vi "pp3_log_sessionParameters.vi"(10 "queue in":refnum<queue>) -> (2 "queue out":refnum<queue>)   [LabVIEW 2013]
uses:
  CTL_pp3c_SessionParam.ctl
panel:
  in  "Session parameters":T1={"Log File Directory Root"=path "E:/Data/SPP.Coulb1", "Subject Name"="SPP074", "Tone repeat (ms)"=0, "Habit tr0 (s)"=180, "ITI min\n(s)"=6, "ITI max\n(s)"=16, "Stay \n(s)"=3, "Run"=TRUE, "Jump time\n(s)"=4, "Start trial"=0, "Log File Directory"=path "E:/Data/SPP.Coulb1/SPP074/161224/161555", "Shock \ndur (s)"=6, "Pre click \n(V)"=0.1, "Click\ndel (s)"=1.0, "Reward CR"=FALSE} {"Click\ndel (s)" min=0.0 step=1.0; "Pre click \n(V)" min=0.0 max=1.0 step=1.0; "Shock \ndur (s)" min=0 step=1; "Stay \n(s)" min=0 step=1; "Start trial" step=1; "Jump time\n(s)" min=0 step=1; "Tone repeat (ms)" min=0 max=1000 step=1; "ITI min\n(s)" min=0 step=1; "ITI max\n(s)" min=0 step=1; "Habit tr0 (s)" min=0 step=1}
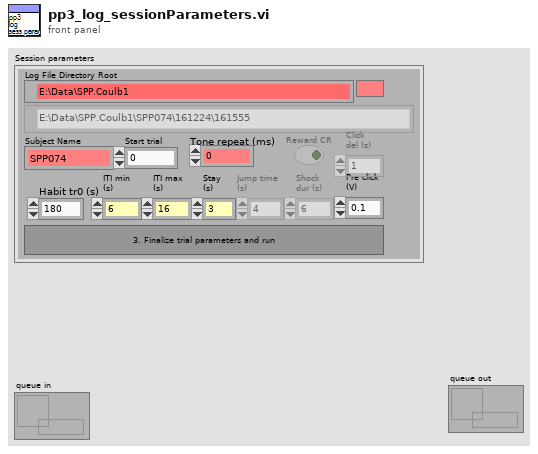
[diagram p1: front panel]
types:
  T1 = typedef "CTL_pp3c_SessionParam.ctl" = cluster{"Log File Directory Root":path, "Subject Name":string, "Tone repeat (ms)":i32, "Habit tr0 (s)":i32, "ITI min\n(s)":i32, "ITI max\n(s)":i32, "Stay \n(s)":i32, "Run":bool, "Jump time\n(s)":i32, "Start trial":u16, "Log File Directory":path, "Shock \ndur (s)":i32, "Pre click \n(V)":dbl, "Click\ndel (s)":dbl, "Reward CR":bool}
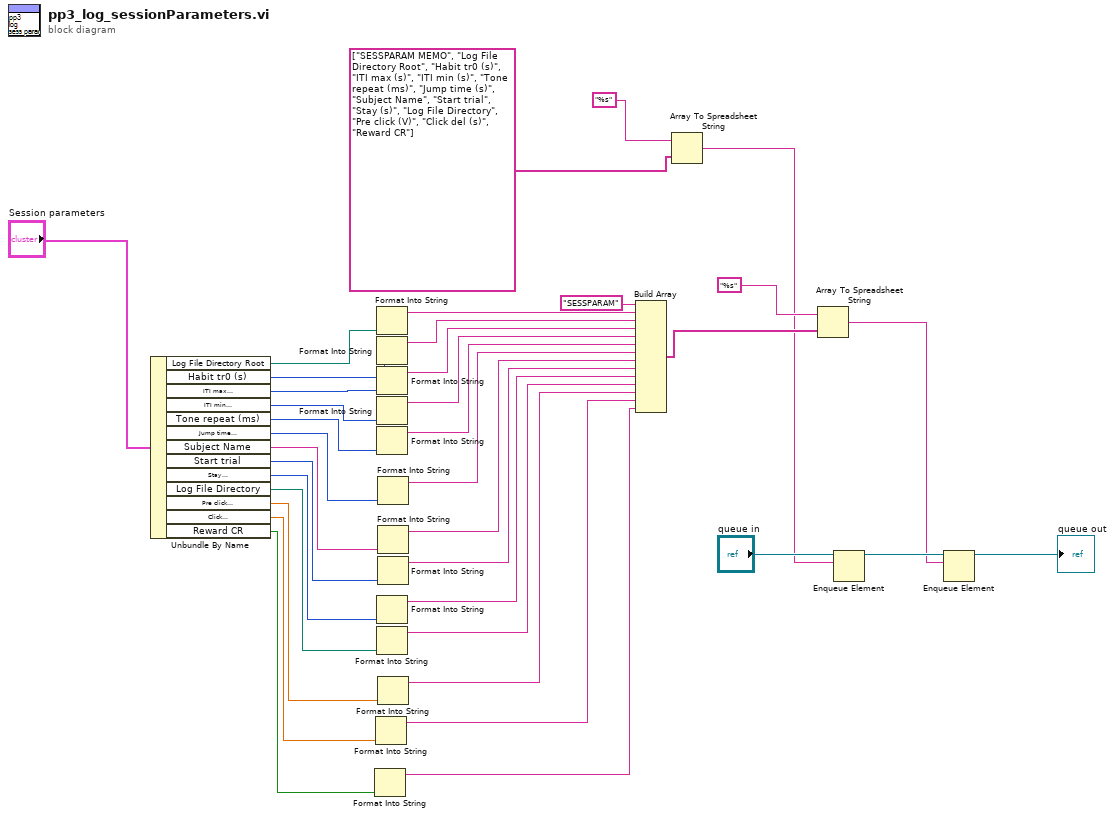
[diagram p0: block diagram]
diagram:
  n1 = Unbundle By Name("Session parameters") -> ("Log File Directory Root"=w37:path, "Habit tr0 (s)"=w34:i32, "ITI max\n(s)"=w33:i32, "ITI min\n(s)"=w32:i32, "Tone repeat (ms)"=w31:i32, "Jump time\n(s)"=w30:i32, "Subject Name"=w24:string, "Start trial"=w23:u16, "Stay \n(s)"=w22:i32, "Log File Directory"=w21:path, "Pre click \n(V)"=w20:dbl, "Click\ndel (s)"=w12:dbl, "Reward CR"=w3:bool)
  n2 = Format Into String(w3) -> (resulting string=w2:string)  [unwired: 3 in, 1 out]
  n3 = Format Into String(w12) -> (resulting string=w11:string)  [unwired: 3 in, 1 out]
  n4 = Format Into String(w37) -> (resulting string=w36:string)  [unwired: 3 in, 1 out]
  n5 = Format Into String(w34) -> (resulting string=w29:string)  [unwired: 3 in, 1 out]
  n6 = Format Into String(w33) -> (resulting string=w28:string)  [unwired: 3 in, 1 out]
  n7 = Format Into String(w32) -> (resulting string=w27:string)  [unwired: 3 in, 1 out]
  n8 = Format Into String(w31) -> (resulting string=w26:string)  [unwired: 3 in, 1 out]
  n9 = Format Into String(w22) -> (resulting string=w17:string)  [unwired: 3 in, 1 out]
  n10 = Format Into String(w21) -> (resulting string=w16:string)  [unwired: 3 in, 1 out]
  n11 = Format Into String(w30) -> (resulting string=w25:string)  [unwired: 3 in, 1 out]
  n12 = Format Into String(w24) -> (resulting string=w19:string)  [unwired: 3 in, 1 out]
  n13 = Format Into String(w23) -> (resulting string=w18:string)  [unwired: 3 in, 1 out]
  n14 = Format Into String(w20) -> (resulting string=w15:string)  [unwired: 3 in, 1 out]
  n15 = Build Array("SESSPARAM" ("element"), w36, w29, w28, w27, w26, w25, w19, w18, w17, w16, w15, w11, w2) -> (w13:string[])
  n16 = Array To Spreadsheet String(array=string[] ["SESSPARAM MEMO", "Log File Directory Root", "Habit tr0 (s)", "ITI max (s)", "ITI min (s)", "Tone repeat (ms)", "Jump time (s)", "Subject Name", "Start trial", "Stay (s)", "Log File Directory", "Pre click (V)", "Click del (s)", "Reward CR"], 3:"%s" ("format string")) -> (spreadsheet string=w5:string)  [unwired: 1 in]
  n17 = Array To Spreadsheet String(array=w13, 3:"%s" ("format string")) -> (spreadsheet string=w4:string)  [unwired: 1 in]
  n18 = Enqueue Element(queue="queue in", element=w5) -> (queue out=w7:refnum<queue>)  [unwired: 2 in, 2 out]
  n19 = Enqueue Element(queue=w7, element=w4) -> (queue out=→"queue out":refnum<queue>)  [unwired: 2 in, 2 out]
